vi "Test ACME Value Extension.vi"() -> ()   [LabVIEW 2013]
uses:
  classes/Test/Test.lvclass
  Assert.ACME.lvclass
panel:
  out "error out":errorcluster
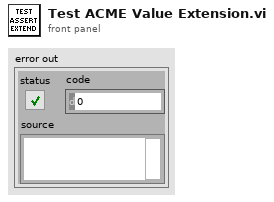
[diagram p1: front panel]
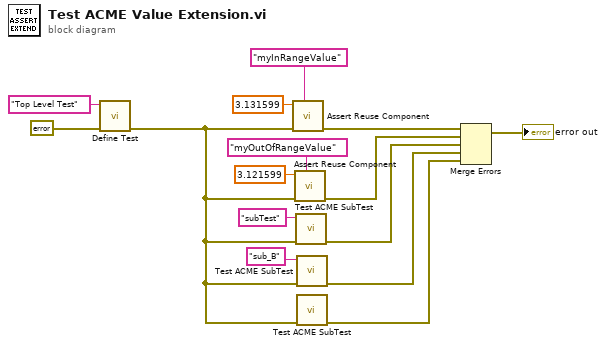
[diagram p0: block diagram]
diagram:
  n1 = call "Define Test.vi"("error in (no error)"=errorcluster {"status"=FALSE, "code"=0, "source"=""}, "Label (VI Title)"="Top Level Test") -> ("error out"=w3:errorcluster)  [unwired: 8 in, 1 out]
  n2 = call "Assert Reuse Component.vi"("Label"="myInRangeValue" ("Label (VI Title)"), "error in (no error)"=w3, "ACME Value"=3.131599) -> ("error out"=w14:errorcluster)  [unwired: 8 in]
  n3 = call "Assert Reuse Component.vi"("Label"="myOutOfRangeValue" ("Label (VI Title)"), "error in (no error)"=w3, "ACME Value"=3.121599) -> ("error out"=w9:errorcluster)  [unwired: 8 in]
  n4 = call "Test ACME SubTest.vi"("error in (no error)"=w3, "Label (VI Title)"="subTest") -> ("error out"=w6:errorcluster)  [unwired: 9 in]
  n5 = call "Test ACME SubTest.vi"("error in (no error)"=w3, "Label (VI Title)"="sub_B") -> ("error out"=w5:errorcluster)  [unwired: 9 in]
  n6 = call "Test ACME SubTest.vi"("error in (no error)"=w3) -> ("error out"=w4:errorcluster)  [unwired: 10 in]
  n7 = Merge Errors(w14, w9, w6, w5, w4) -> (→"error out":errorcluster)
